vi "脉冲参数检查.vi"(7 "队列输入":refnum<queue>, 8 "NewVal输入":T1 {"测试参数"."反向极限电流(mA)" min=0.0 max=3000.0; "测试参数"."反向电压(V)" min=0.0 max=40.0; "测试参数"."读取电压(V)" min=0.0 max=40.0; "测试参数"."正向极限电流(mA)" min=0.0 max=3000.0; "测试参数"."正向电压(V)" min=0.0 max=40.0}, 11 "错误输入（无错误）":errorcluster) -> (0 "NewVal输出":T1 {"测试参数"."反向极限电流(mA)" min=0.0 max=3000.0; "测试参数"."反向电压(V)" min=0.0 max=40.0; "测试参数"."读取电压(V)" min=0.0 max=40.0; "测试参数"."正向极限电流(mA)" min=0.0 max=3000.0; "测试参数"."正向电压(V)" min=0.0 max=40.0}, 3 "错误输出":errorcluster)   [LabVIEW 2021]
uses:
  QueueLib/QueueLib.lvlib
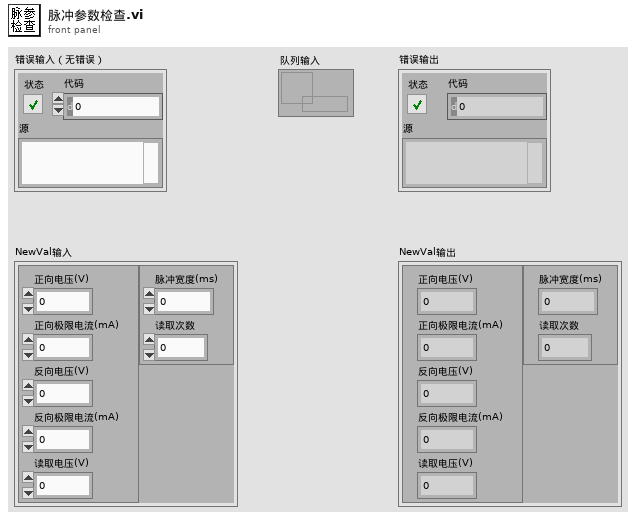
[diagram p1: front panel]
types:
  T1 = typedef "脉冲参数.ctl" = cluster{"测试参数":cluster{"正向电压(V)":dbl, "正向极限电流(mA)":dbl, "反向电压(V)":dbl, "反向极限电流(mA)":dbl, "读取电压(V)":dbl}, "时序参数":cluster{"脉冲宽度(ms)":dbl, "读取次数":u32}}
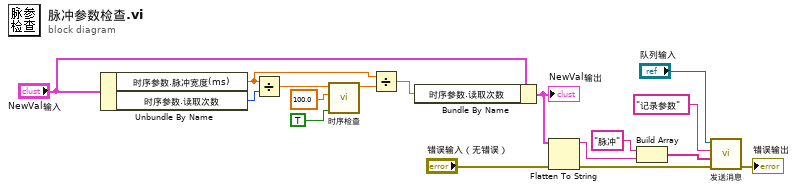
[diagram p0: block diagram]
diagram:
  n1 = Unbundle By Name("NewVal输入") -> ("时序参数.脉冲宽度(ms)"=w13:dbl, "时序参数.读取次数"=w9:u32)
  n2 = Divide(x=w13, y=w9) -> (x/y=w10:dbl)
  n3 = call "时序检查.vi"("时序优先"=TRUE, "nplc"=100.0, "测量间隔"=w10) -> ("测量间隔输出"=w14:dbl)  [unwired: 7 in, 1 out]
  n4 = Divide(x=w13, y=w14) -> (x/y=w15:dbl)
  n5 = Bundle By Name(cluster="NewVal输入", "时序参数.读取次数"=w15) -> (w17:T1)
  "NewVal输出" <- w17
  n6 = Flatten To String(anything=w17, error in (no error)="错误输入（无错误）") -> (data string=w3:string, error out=w1:errorcluster)  [unwired: 2 in, 1 out]
  n7 = Build Array("脉冲" ("元素"), w3) -> (w5:string[])
  n8 = call "发送消息.vi"("错误输入（无错误）"=w1, "数据"=w5, "消息"="记录参数", "输入队列"="队列输入") -> ("错误输出"=→"错误输出":errorcluster)  [unwired: 6 in, 1 out]
